vi "Search 2D Array (U16).vi"(10 "Element":u16, 11 "Array":u16[][](array[numeric])) -> (3 "Locations":i32[][](array[numeric]))   [LabVIEW 2020]
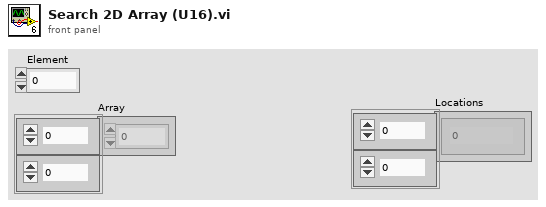
[diagram p1: front panel]
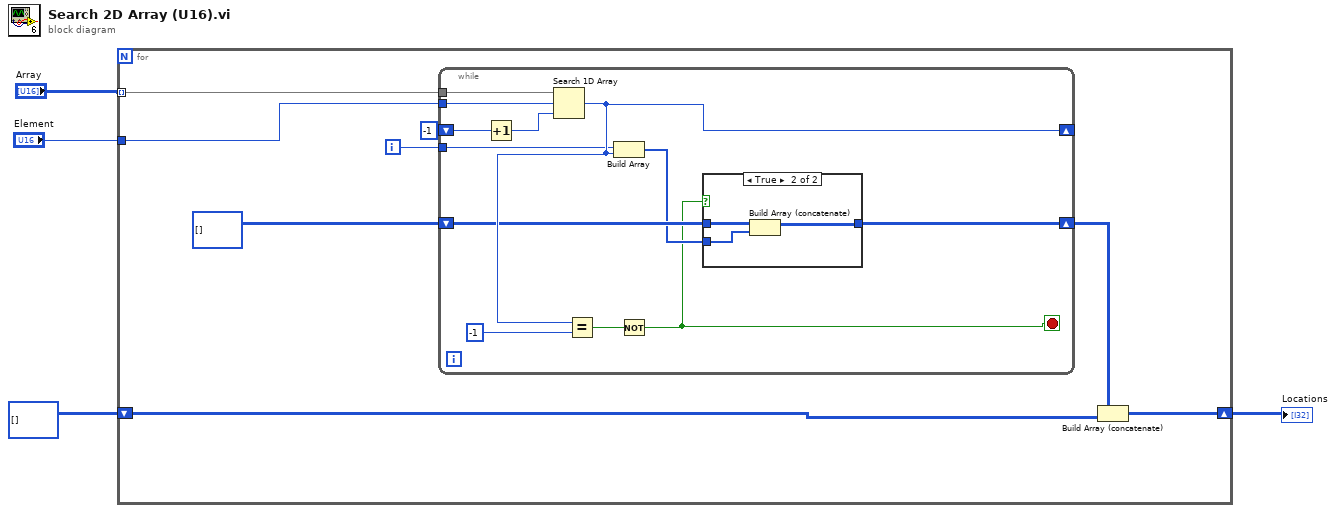
[diagram p0: block diagram]
diagram:
  n1 = for {
    tunnel: "Array" -> [w12] mode=indexing
    tunnel: "Element" -> [w11]
    shift-right: [w8] -> w3
    shift-left: i32[][] [] -> [w6]
    i -> [w10]
    n2 = while {
      tunnel: w12 -> [w24]
      tunnel: w11 -> [w23]
      shift-right: [w20] -> _
      shift-left: -1 ("index of element") -> [w22]
      tunnel: w10 -> [w19]
      shift-right: [w16] -> w5
      shift-left: i32[][] [] ("Array 2") -> [w17]
      stop <- w13 stop-if-true
      n3 = Increment(x=w22) -> (x+1=w18:i32)
      n4 = Search 1D Array(1D array=w24, element=w23, start index (0)=w18) -> (index of element=w20:i32)
      n5 = Equal?(x=w20, y=-1) -> (x = y?=w14:bool)
      n6 = Build Array(w19, w20) -> (w15:i32[])
      n7 = Not(x=w14) -> (.not. x?=w13:bool)
      n8 = case shown="True" w13 {
        tunnel: w17 -> [w25 w27]
        tunnel: w15 -> [_ w26]
        tunnel: [w25 w28] -> w16
        frame False {
        }
        frame True {
          n9 = Build Array (concatenate)(w27, w26) -> (w28:i32[][])
        }
      }
    }
    n10 = Build Array (concatenate)(w5, w6) -> (w8:i32[][])
  }
  "Locations" <- w3
